vi "Enter.vi"(8 "error in (no error)":errorcluster, 11 "Room in":refnum<class "Room.lvclass">) -> (0 "error out":errorcluster, 3 "Room out":refnum<class "Room.lvclass">)   [LabVIEW 2020, in "Room.lvclass"]
uses:
  Room.lvclass
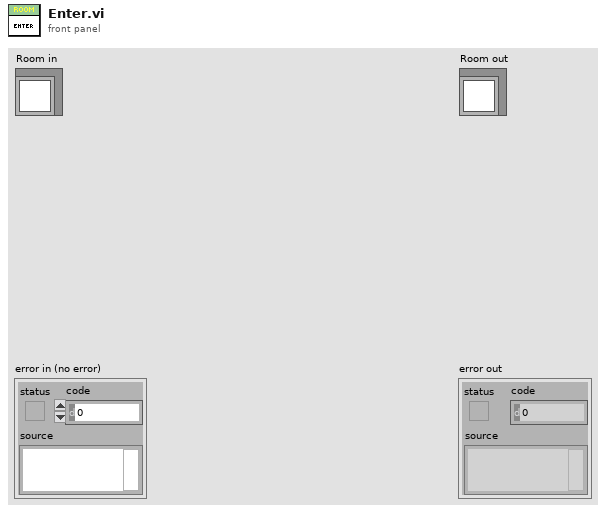
[diagram p1: front panel]
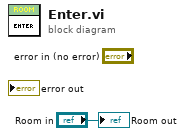
[diagram p0: block diagram]
diagram:
  "Room out" <- "Room in"
